vi "Bo Peep Begin.vi"   [LabVIEW 2014]
uses:
  <vilib>/Rock Robotics/SystemInterfaces/AI/FPGA_AIChannel.ctl
  <vilib>/Rock Robotics/WPI/Ultrasonic/WPI_SonarMB1010AnalogOpen.vi
  <vilib>/Rock Robotics/WPI/Ultrasonic/WPI_SonarMB1010AnalogRefNum Registry Set.vi
  Robot Global Data.vi
types:
  T1 = typedef "FPGA_AIChannel.ctl" = enum8{"AI 0", "AI 1", "AI 2", "AI 3", "AI MXP 0", "AI MXP 1", "AI MXP 2", "AI MXP 3", "Invalid"}
  T2 = typedef "WPI_SonarMB1010AnalogDeviceRef.ctl" = cluster{"AIDeviceRef":T3, "Scaling factor (V/in)":dbl, "Average Bits":u8}
  T3 = typedef "WPI_AnalogChannelDevRef.ctl" = cluster{"DevStatus":errorcluster, "Controller":T4, "Analog Channel":T1}
  T4 = typedef "FPGA_TypedefAnalogModule.ctl" = enum16{"Controller 1"}
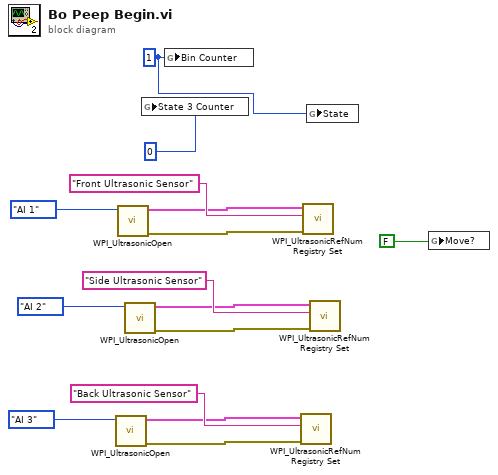
[diagram p0: block diagram]
diagram:
  w2 = i8 1 ("Bin Counter")
  n1 = call-poly <vilib>:"WPI_UltrasonicOpen.vi"("Analog Channel"=FPGA_AIChannel."AI 3") -> ("error out"=w12:errorcluster, "SonarMB1010AnalogDevRef"=w13:T2)  [unwired: 9 in]
  n2 = call-poly <vilib>:"WPI_UltrasonicOpen.vi"("Analog Channel"=FPGA_AIChannel."AI 1") -> ("error out"=w4:errorcluster, "SonarMB1010AnalogDevRef"=w5:T2)  [unwired: 9 in]
  n3 = call-poly <vilib>:"WPI_UltrasonicOpen.vi"("Analog Channel"=FPGA_AIChannel."AI 2") -> ("error out"=w8:errorcluster, "SonarMB1010AnalogDevRef"=w9:T2)  [unwired: 9 in]
  n4 = global write "Robot Global Data.vi" "State 3 Counter"(i8 0 ("State")) -> ()
  n5 = global write "Robot Global Data.vi" "Bin Counter"(w2) -> ()
  n6 = call-poly <vilib>:"WPI_UltrasonicRefNum Registry Set.vi"("error in (no error)"=w12, "refnum name"="Back Ultrasonic Sensor", "SonarMB1010AnalogDevRef"=w13) -> ()  [unwired: 7 in, 2 out]
  n7 = call-poly <vilib>:"WPI_UltrasonicRefNum Registry Set.vi"("error in (no error)"=w4, "refnum name"="Front Ultrasonic Sensor", "SonarMB1010AnalogDevRef"=w5) -> ()  [unwired: 7 in, 2 out]
  n8 = global write "Robot Global Data.vi" "State"(w2) -> ()
  n9 = call-poly <vilib>:"WPI_UltrasonicRefNum Registry Set.vi"("error in (no error)"=w8, "refnum name"="Side Ultrasonic Sensor", "SonarMB1010AnalogDevRef"=w9) -> ()  [unwired: 7 in, 2 out]
  n10 = global write "Robot Global Data.vi" "Move?"(FALSE) -> ()
